vi "load last configuration.vi"(8 "error in (no error)":errorcluster, 10 "name or relative path":string="last configuration.ini", 11 "base path":path) -> (0 "error out":errorcluster)   [LabVIEW 2015]
uses:
  <vilib>/Utility/config.llb/Read Key (String).vi
  global variables/params.vi
  <vilib>/Utility/config.llb/NI_LVConfig.lvlib
panel:
  out "appended path":path
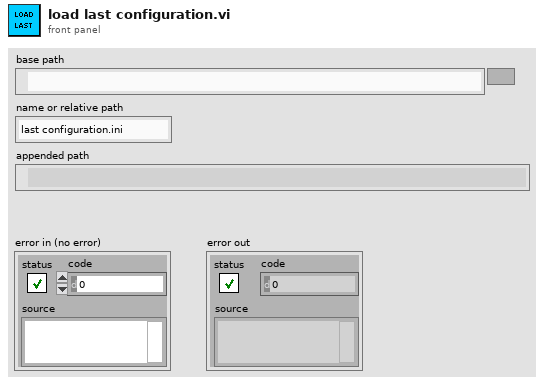
[diagram p1: front panel]
types:
  T1 = typedef "NI_LVConfig.lvlib/Config Data RefNum.ctl" = refnum<k1>
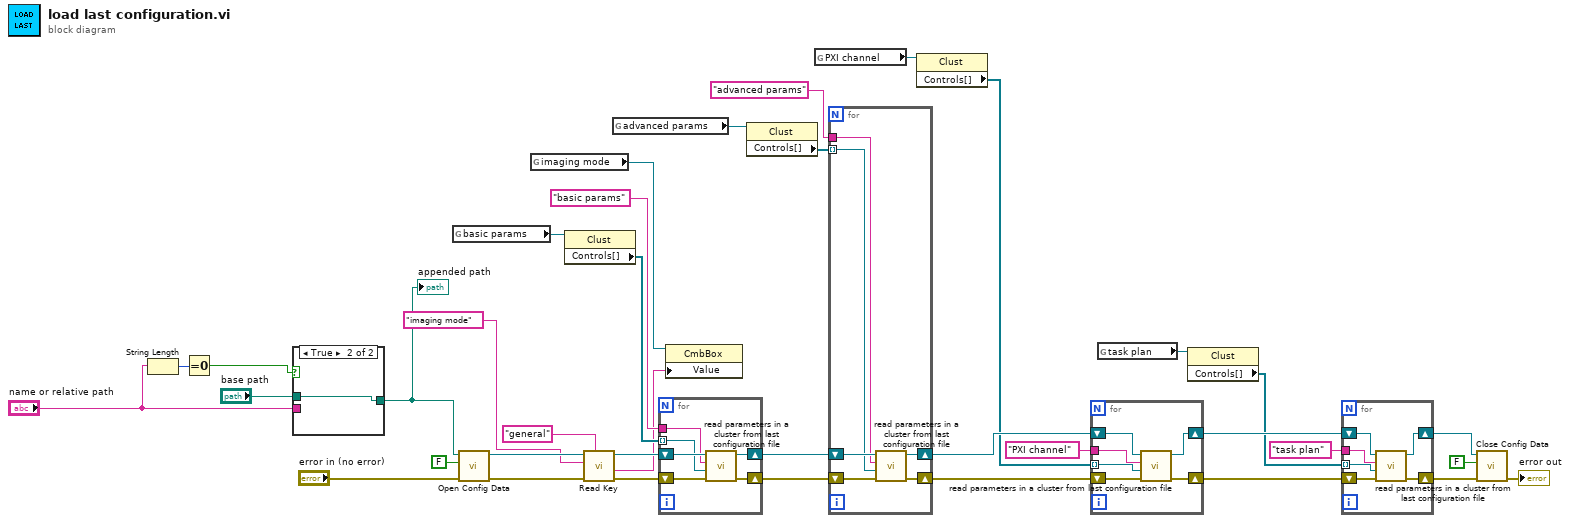
[diagram p0: block diagram]
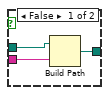
[diagram p2: hidden frame]
diagram:
  n1 = String Length(string="name or relative path") -> (length=w5:i32)
  n2 = Equal To 0?(x=w5) -> (x = 0?=w4:bool)
  n3 = case shown="True" w4 {
    tunnel: "name or relative path" -> [w38 _]
    tunnel: "base path" -> [w39 w41]
    tunnel: [w40 w41] -> w1
    frame False {
      n4 = Build Path(base path=w39, name or relative path=w38) -> (appended path=w40:path)
    }
    frame True {
    }
  }
  "appended path" <- w1
  n5 = global read "params.vi" "basic params"() -> (w19:refnum<vi>)
  n6 = call <vilib>:"Open Config Data.vi"("error in (no error)"="error in (no error)", "create file if necessary (T)"=FALSE, "configuration file path"=w1) -> ("error out"=w28:errorcluster, "refnum"=w31:T1)  [unwired: 6 in, 1 out]
  n7 = global read "params.vi" "imaging mode"() -> (w20:refnum<vi>)
  n8 = property class="Clust"(reference=w19) -> ("Controls[]"=w23:refnum<vi>[])  [unwired: 1 in, 2 out]
  n9 = call-poly <vilib>:"Read Key.vi"("section"="general", "error in (no error)"=w28, "key"="imaging mode", "refnum"=w31) -> ("error out"=w29:errorcluster, "value"=w21:string, "refnum out"=w30:T1)  [unwired: 4 in, 1 out]
  n10 = global read "params.vi" "advanced params"() -> (w18:refnum<vi>)
  n11 = for {
    tunnel: w23 -> [w45] mode=indexing
    tunnel: "basic params" -> [w46]
    shift-right: [w42] -> w25
    shift-left: w30 -> [w47]
    shift-right: [w43] -> w24
    shift-left: w29 -> [w44]
    n12 = call "read parameters in a cluster from last configuration file.vi"("error in (no error)"=w44, "Control in"=w45, "section"=w46, "refnum in"=w47) -> ("error out"=w43:errorcluster, "Refnum out"=w42:T1)  [unwired: 6 in]
  }
  n13 = property class="CmbBox"(reference=w20, "Value"=w21) -> ()  [unwired: 1 in, 2 out]
  n14 = property class="Clust"(reference=w18) -> ("Controls[]"=w22:refnum<vi>[])  [unwired: 1 in, 2 out]
  n15 = global read "params.vi" "PXI channel"() -> (w14:refnum<vi>)
  n16 = for {
    tunnel: w22 -> [w51] mode=indexing
    tunnel: "advanced params" -> [w52]
    shift-right: [w49] -> w15
    shift-left: w25 -> [w53]
    shift-right: [w48] -> w16
    shift-left: w24 -> [w50]
    n17 = call "read parameters in a cluster from last configuration file.vi"("error in (no error)"=w50, "Control in"=w51, "section"=w52, "refnum in"=w53) -> ("error out"=w48:errorcluster, "Refnum out"=w49:T1)  [unwired: 6 in]
  }
  n18 = property class="Clust"(reference=w14) -> ("Controls[]"=w13:refnum<vi>[])  [unwired: 1 in, 2 out]
  n19 = for {
    tunnel: w13 -> [w57] mode=indexing
    tunnel: "PXI channel" -> [w58]
    shift-right: [w55] -> w10
    shift-left: w15 -> [w59]
    shift-right: [w54] -> w12
    shift-left: w16 -> [w56]
    n20 = call "read parameters in a cluster from last configuration file.vi"("error in (no error)"=w56, "Control in"=w57, "section"=w58, "refnum in"=w59) -> ("error out"=w54:errorcluster, "Refnum out"=w55:T1)  [unwired: 6 in]
  }
  n21 = global read "params.vi" "task plan"() -> (w7:refnum<vi>)
  n22 = property class="Clust"(reference=w7) -> ("Controls[]"=w6:refnum<vi>[])  [unwired: 1 in, 2 out]
  n23 = for {
    shift-right: [w62] -> w11
    shift-left: w12 -> [w63]
    shift-right: [w64] -> w9
    shift-left: w10 -> [w65]
    tunnel: "task plan" ("section") -> [w61]
    tunnel: w6 -> [w60] mode=indexing
    n24 = call "read parameters in a cluster from last configuration file.vi"("error in (no error)"=w63, "Control in"=w60, "section"=w61, "refnum in"=w65) -> ("error out"=w62:errorcluster, "Refnum out"=w64:T1)  [unwired: 6 in]
  }
  n25 = call <vilib>:"Close Config Data.vi"("error in (no error)"=w11, "write file if changed (T)"=FALSE, "refnum"=w9) -> ("error out"=→"error out":errorcluster)  [unwired: 7 in, 1 out]
